vi "TSM SSC DCPower Filter Pins.vi"(0 "DCPower TSM in":T1, 5 "Requested Pins":tag[](array[tag]), 11 "error in":errorcluster) -> (4 "Filtered DCPower TSM out":T1, 15 "error out":errorcluster)   [LabVIEW 2020]
doc: "This VI filters the TSM SSC cluster to requested pins."
uses:
  TSM SSC DCPower.ctl
  <vilib>/NI_TestStand_SemiconductorModule/NI_TestStand_Semiconductor_Module.lvlibp/PinMap/PinQueryContext/MultiplePinMultipleSessionQueryContext/MultiplePinMultipleSessionQueryContext.lvclass
  SSC DCPower/SSC DCPower.ctl
  Shared SubVIs/TSM Pin Abstraction/TSM Pin Information.ctl
  Shared SubVIs/TSM Pin Abstraction/TSM Pin Type Identifier.ctl
  Shared SubVIs/TSM Pin Abstraction/TSM Expanded Pin Information.ctl
  Shared SubVIs/Channel List to Pins.vi
  Shared SubVIs/Trim Whitespace [Inlined].vi
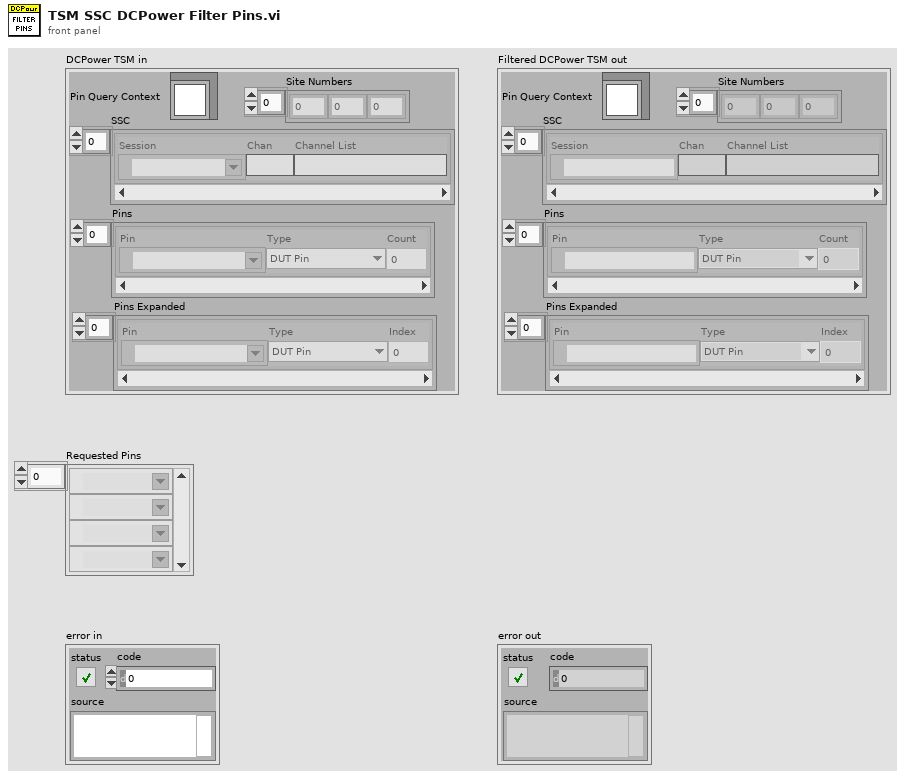
[diagram p1: front panel]
types:
  T1 = typedef "TSM SSC DCPower.ctl" = cluster{"Pin Query Context":refnum<class "MultiplePinMultipleSessionQueryContext.lvclass">, "SSC":T2[], "Site Numbers":i32[], "Pins":T3[], "Pins Expanded":T5[]}
  T2 = typedef "SSC DCPower.ctl" = cluster{"Session":refnum<k15>, "Chan":string, "Channel List":string}
  T3 = typedef "TSM Pin Information.ctl" = cluster{"Pin":tag, "Type":T4, "Count":i32}
  T4 = typedef "TSM Pin Type Identifier.ctl" = enum8{"DUT Pin", "System Pin", "Pin Group", "Not Determined"}
  T5 = typedef "TSM Expanded Pin Information.ctl" = cluster{"Pin":tag, "Type":T4, "Index":i32}
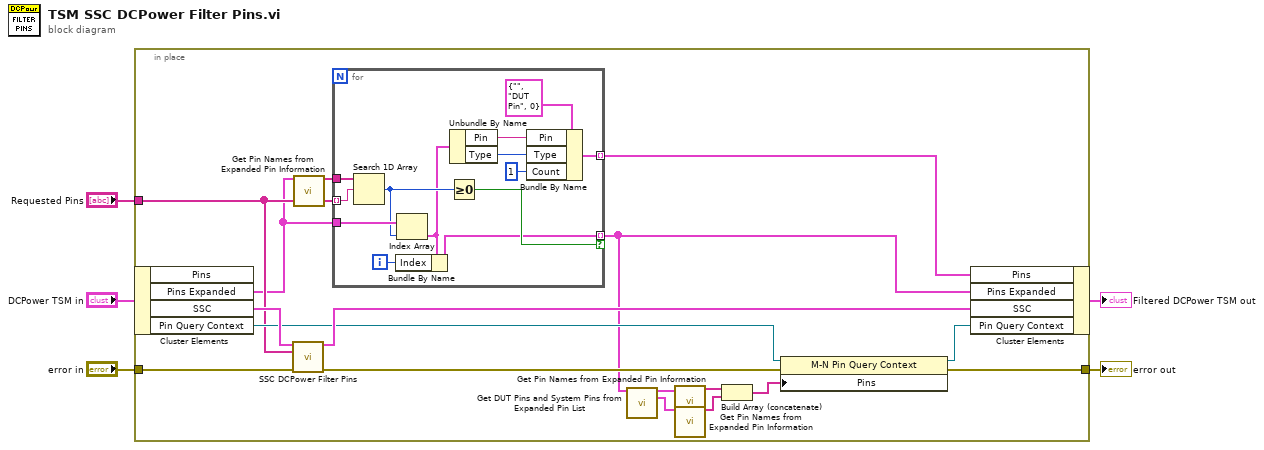
[diagram p0: block diagram]
diagram:
  n1 = in-place {
    in-place-border: "Requested Pins" -> [w18]
    in-place-border: "error in" -> [w13]
    in-place-border: [w12] -> w1
    n2 = in-place-cluster #1("DCPower TSM in") -> ("Pins Expanded"=w17:T5[], "SSC"=w22:T2[], "Pin Query Context"=w20:refnum<class "MultiplePinMultipleSessionQueryContext.lvclass">)  [unwired: 1 out]
    n3 = call "SSC DCPower Filter Pins.vi"("DCPower SSC in"=w22, "Requested Pins"=w18, "error in"=w13) -> ("Filtered DCPower SSC out"=w21:T2[], "error out"=w14:errorcluster)  [unwired: 11 in]
    n4 = call "Get Pin Names from Expanded Pin Information.vi"("Expanded Pin Information"=w17) -> ("Pins"=w16:tag[])  [unwired: 14 in]
    n5 = for {
      tunnel: w17 -> [w32]
      tunnel: w18 -> [w33] mode=indexing
      tunnel: [w24] -> w11 mode=indexing if=w35
      tunnel: w16 -> [w34]
      tunnel: [w25] -> w15 mode=indexing
      i -> [w23]
      n6 = Search 1D Array(1D array=w34, element=w33) -> (index of element=w31:i32)  [unwired: 1 in]
      n7 = Index Array(array=w32, index=w31) -> (element=w29:T5)
      n8 = Bundle By Name(cluster=w29, "Index"=w23) -> (w24:T5)
      n9 = Greater Or Equal To 0?(x=w31) -> (x >= 0?=w35:bool)
      n10 = Unbundle By Name(w29) -> ("Pin"=w28:tag, "Type"=w27:T4)
      n11 = Bundle By Name(cluster=T3 {"Pin"="", "Type"=enum."DUT Pin", "Count"=0} ("Pin Information"), "Pin"=w28, "Type"=w27, "Count"=1) -> (w25:T3)
    }
    n12 = call "Get DUT Pins and System Pins from Expanded Pin List.vi"("Expanded Pin Information"=w11) -> ("DUT Pins"=w10:T5[], "System Pins"=w9:T5[])  [unwired: 13 in]
    n13 = call "Get Pin Names from Expanded Pin Information.vi"("Expanded Pin Information"=w10) -> ("Pins"=w8:tag[])  [unwired: 14 in]
    n14 = call "Get Pin Names from Expanded Pin Information.vi"("Expanded Pin Information"=w9) -> ("Pins"=w6:tag[])  [unwired: 14 in]
    n15 = Build Array (concatenate)(w8, w6) -> (w7:tag[])
    n16 = property class="M-N Pin Query Context"(reference=w20, error in=w14, "Pins"=w7) -> (reference out=w19:refnum<class "MultiplePinMultipleSessionQueryContext.lvclass">, error out=w12:errorcluster)
    n17 = in-place-cluster #1("Pins"=w15, "Pins Expanded"=w11, "SSC"=w21, "Pin Query Context"=w19) -> (→"Filtered DCPower TSM out":T1)
  }
  "error out" <- w1
